vi "MicroPulse data length.vi"(2 "count length":i32, 3 "[U8] count bytes":u8[](array[numeric])) -> (0 "total msg length":i32, 1 "data length":i32)   [LabVIEW 2026, in "MicroPulse_Driver.lvlib"]
uses:
  MicroPulse_Driver.lvlib
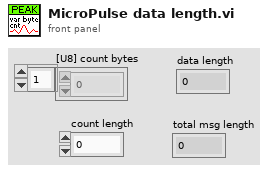
[diagram p1: front panel]
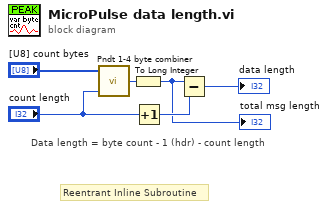
[diagram p0: block diagram]
diagram:
  # "Reentrant Inline Subroutine"
  # "Data length = byte count - 1 (hdr) - count length"
  n1 = call "Pndt 1-4 byte combiner.vi"("#bytes"="count length", "[U8] count bytes"="[U8] count bytes") -> ("U32"=w3:u32)  [unwired: 1 in]
  n2 = To Long Integer(number=w3) -> (32bit integer=w1:i32)
  "total msg length" <- w1
  n3 = Increment(x="count length") -> (x+1=w5:i32)
  n4 = Subtract(x=w1, y=w5) -> (x-y=→"data length":i32)
